vi "write_dac2_command.vi"(10 "dac2 voltage":dbl, 11 "dac2 toggle":bool) -> (2 "Command Out":string)   [LabVIEW 2015]
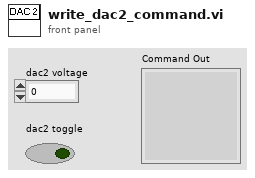
[diagram p1: front panel]
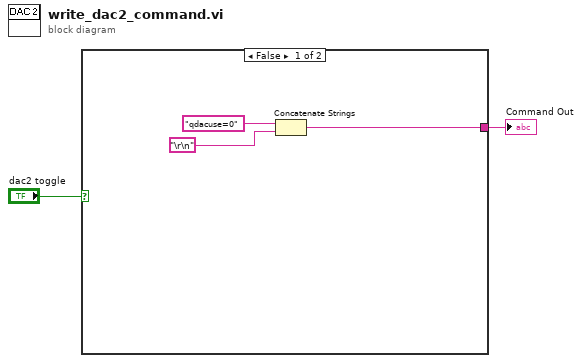
[diagram p0: block diagram]
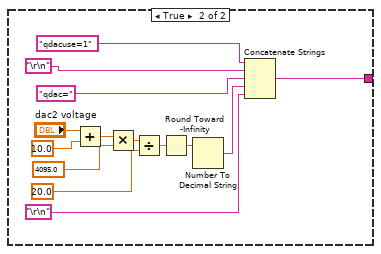
[diagram p2: hidden frame]
diagram:
  n1 = case shown="False" "dac2 toggle" {
    tunnel: [w3 w6] -> w1
    frame False {
      n2 = Concatenate Strings("qdacuse=0", "\r\n") -> (w3:string)
    }
    frame True {
      n3 = Add(x="dac2 voltage", y=10.0) -> (x+y=w14:dbl)
      n4 = Multiply(x=w14, y=4095.0) -> (x*y=w12:dbl)
      n5 = Divide(x=w12, y=20.0) -> (x/y=w10:dbl)
      n6 = Round Toward -Infinity(1:w10) -> (0:w9:dbl)
      n7 = Number To Decimal String(number=w9) -> (decimal integer string=w8:string)  [unwired: 1 in]
      n8 = Concatenate Strings("qdacuse=1", "\r\n", "qdac=", w8, "\r\n") -> (w6:string)
    }
  }
  "Command Out" <- w1
